vi "MD5.vi"(8 "error in (no error)":errorcluster, 11 "Input String":string) -> (0 "error out":errorcluster, 3 "MD5 message-digest":string)   [LabVIEW 2014, in "lvprj2html.lvlib"]
uses:
  lvprj2html.lvlib
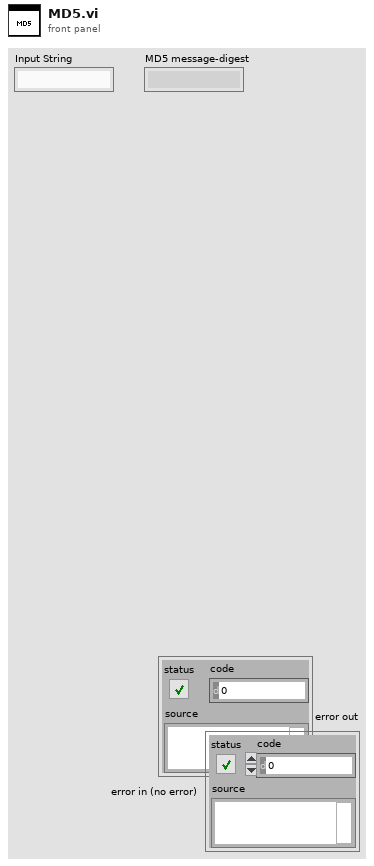
[diagram p1: front panel]
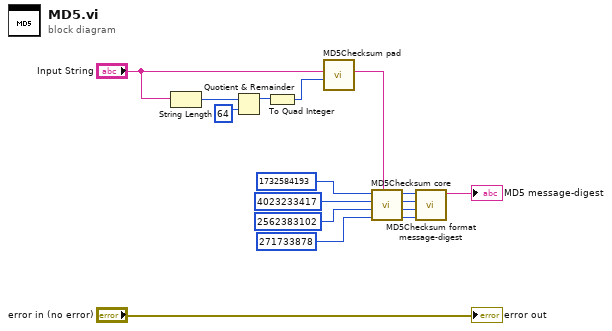
[diagram p0: block diagram]
diagram:
  n1 = String Length(string="Input String") -> (length=w13:i32)
  n2 = Quotient & Remainder(x=w13, y=64) -> (x-y*floor(x/y)=w15:i32)  [unwired: 1 out]
  n3 = To Quad Integer(1:w15) -> (0:w16:i64)
  n4 = call <vilib>:"MD5Checksum pad.vi"("Message String Length (bytes)"=w16, "Last Part of Message String"="Input String") -> ("Padding"=w11:string)  [unwired: 9 in]
  n5 = call <vilib>:"MD5Checksum core.vi"("Input String"=w11, "s4 in"=u32 271733878 ("s4"), "s3 in"=u32 2562383102 ("s3"), "s2 in"=u32 4023233417 ("s2"), "s1 in"=u32 1732584193 ("s1")) -> ("s4 out"=w9:u32, "s3 out"=w8:u32, "s2 out"=w7:u32, "s1 out"=w6:u32)  [unwired: 3 in]
  n6 = call <vilib>:"MD5Checksum format message-digest.vi"("s4"=w9, "s3"=w8, "s2"=w7, "s1"=w6) -> ("MD5 message-digest"=→"MD5 message-digest":string)  [unwired: 7 in]
  "error out" <- "error in (no error)"
